vi "background4.vi"() -> ()   [LabVIEW 2014]
uses:
  cloud.ctl
  heart.ctl
  <vilib>/Utility/inputDevices.llb/keyboardAcquire.vi
  <vilib>/Utility/inputDevices.llb/closeKeyboard.vi
panel:
  out "User 1":T1
  out "User 2":T1
  out "Ring 6":T2
  out "Ring 5":T3
  out "Ring 4":T3
  out "Ring 3":T2
  out "2jump":bool=TRUE
  out "User2 name":string
  out "User1 name":string
  out "人1生命":dbl
  out "人2生命":dbl
  out "heart 6":T4
  out "heart 5":T4
  out "heart 4":T4
  out "heart 3":T4
  out "heart 2":T4
  out "heart 1":T4
  out "雲  3":T5
  out "black hole":T6
  out "雲 2":T5
  out "雲":T5
  out "1jump":bool=TRUE
  out "火右飛 2":bool=TRUE
  out "火左飛 2":bool
  out "火左飛":bool
  out "1":T7
  out "火右飛":bool=TRUE
  out "2":T8
  out "2-1":T7
  out "2-2":T8
  in  "stop jump2":bool
  in  "stop jump1":bool
  out "keys pressed":T9(array[ring])
  in  "right/left 2":bool
  in  "人2":bool
  in  "right/left":bool
  in  "人1":bool
  in  "整個遊戲中止":bool
  # "587"
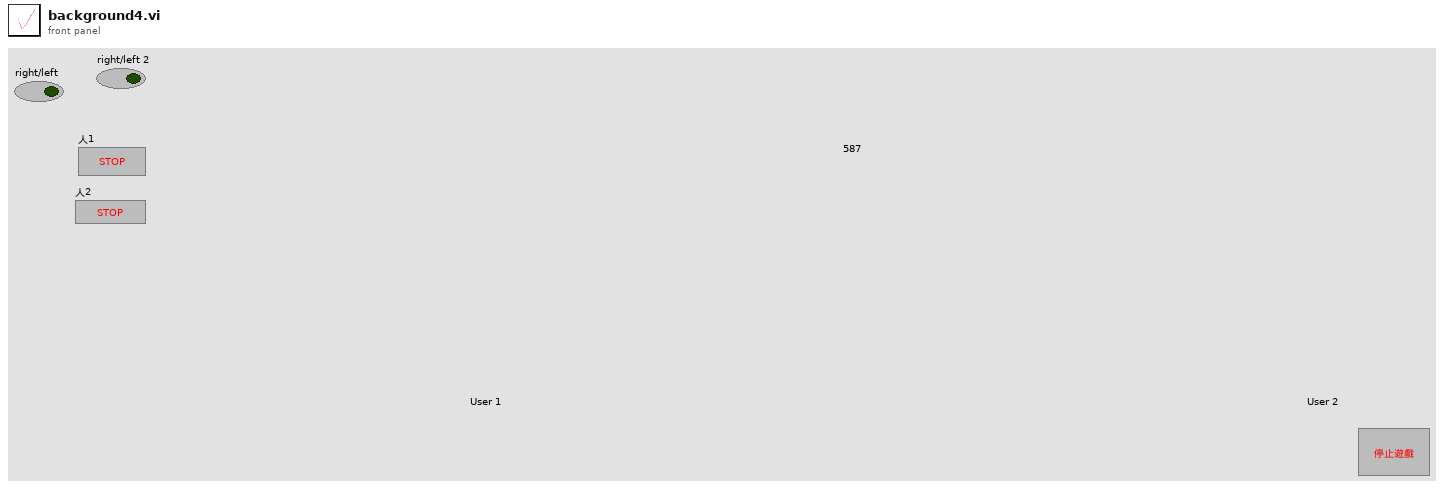
[diagram p1: front panel]
types:
  T1 = typedef "Control 3.ctl" = u16
  T2 = typedef "窄短cloud.ctl" = u16
  T3 = typedef "窄cloud.ctl" = u16
  T4 = typedef "heart.ctl" = u16
  T5 = typedef "cloud.ctl" = u16
  T6 = typedef "Control 4.ctl" = u16
  T7 = typedef "火焰.ctl" = u16
  T8 = typedef "火焰2.ctl" = u16
  T9 = enum16{"0", "1", "2", "3", "4", "5", "6", "7", "8", "9", "A", "B", "C", "D", "E", "F", "G", "H", "I", "J", "K", "L", "M", "N", "O", "P", "Q", "R", "S", "T", "U", "V", "W", "X", "Y", "Z", "F1", "F2", "F3", "F4", "F5", "F6", "F7", "F8", "F9", "F10", "F11", "F12", "F13", "F14", "F15", "ADD", "BACK", "BACKSLASH", "CAPITAL", "COMMA", "DECIMAL", "DELETE", "DIVIDE", "DOWN", "END", "EQUALS", "ESCAPE", "GRAVE (`)", "HOME", "INSERT", "LBRACKET", "LCONTROL", "LEFT", "L ALT", "LSHIFT", "LWIN", "MINUS", "MULTIPLY", "NEXT", "NUMLOCK", "NUMPAD_0", "NUMPAD_1", "NUMPAD_2", "NUMPAD_3", "NUMPAD_4", "NUMPAD_5", "NUMPAD_6", "NUMPAD_7", "NUMPAD_8", "NUMPAD_9", "PAUSE", "PERIOD", "PRIOR (PG UP)", "RBRACKET", "RCONTROL", "RETURN", "RIGHT", "R ALT", "RSHIFT", "RWIN", "SCROLL", "SEMICOLON", "SLASH", "SPACE", "SUBTRACT", "TAB", "UP", "ENTER (num pad)", "' (quote)"}[]
  T10 = enum16{"0", "1", "2", "3", "4", "5", "6", "7", "8", "9", "A", "B", "C", "D", "E", "F", "G", "H", "I", "J", "K", "L", "M", "N", "O", "P", "Q", "R", "S", "T", "U", "V", "W", "X", "Y", "Z", "F1", "F2", "F3", "F4", "F5", "F6", "F7", "F8", "F9", "F10", "F11", "F12", "F13", "F14", "F15", "ADD", "BACK", "BACKSLASH", "CAPITAL", "COMMA", "DECIMAL", "DELETE", "DIVIDE", "DOWN", "END", "EQUALS", "ESCAPE", "GRAVE (`)", "HOME", "INSERT", "LBRACKET", "LCONTROL", "LEFT", "L ALT", "LSHIFT", "LWIN", "MINUS", "MULTIPLY", "NEXT", "NUMLOCK", "NUMPAD_0", "NUMPAD_1", "NUMPAD_2", "NUMPAD_3", "NUMPAD_4", "NUMPAD_5", "NUMPAD_6", "NUMPAD_7", "NUMPAD_8", "NUMPAD_9", "PAUSE", "PERIOD", "PRIOR (PG UP)", "RBRACKET", "RCONTROL", "RETURN", "RIGHT", "R ALT", "RSHIFT", "RWIN", "SCROLL", "SEMICOLON", "SLASH", "SPACE", "SUBTRACT", "TAB", "UP", "ENTER (num pad)", "' (quote)"}
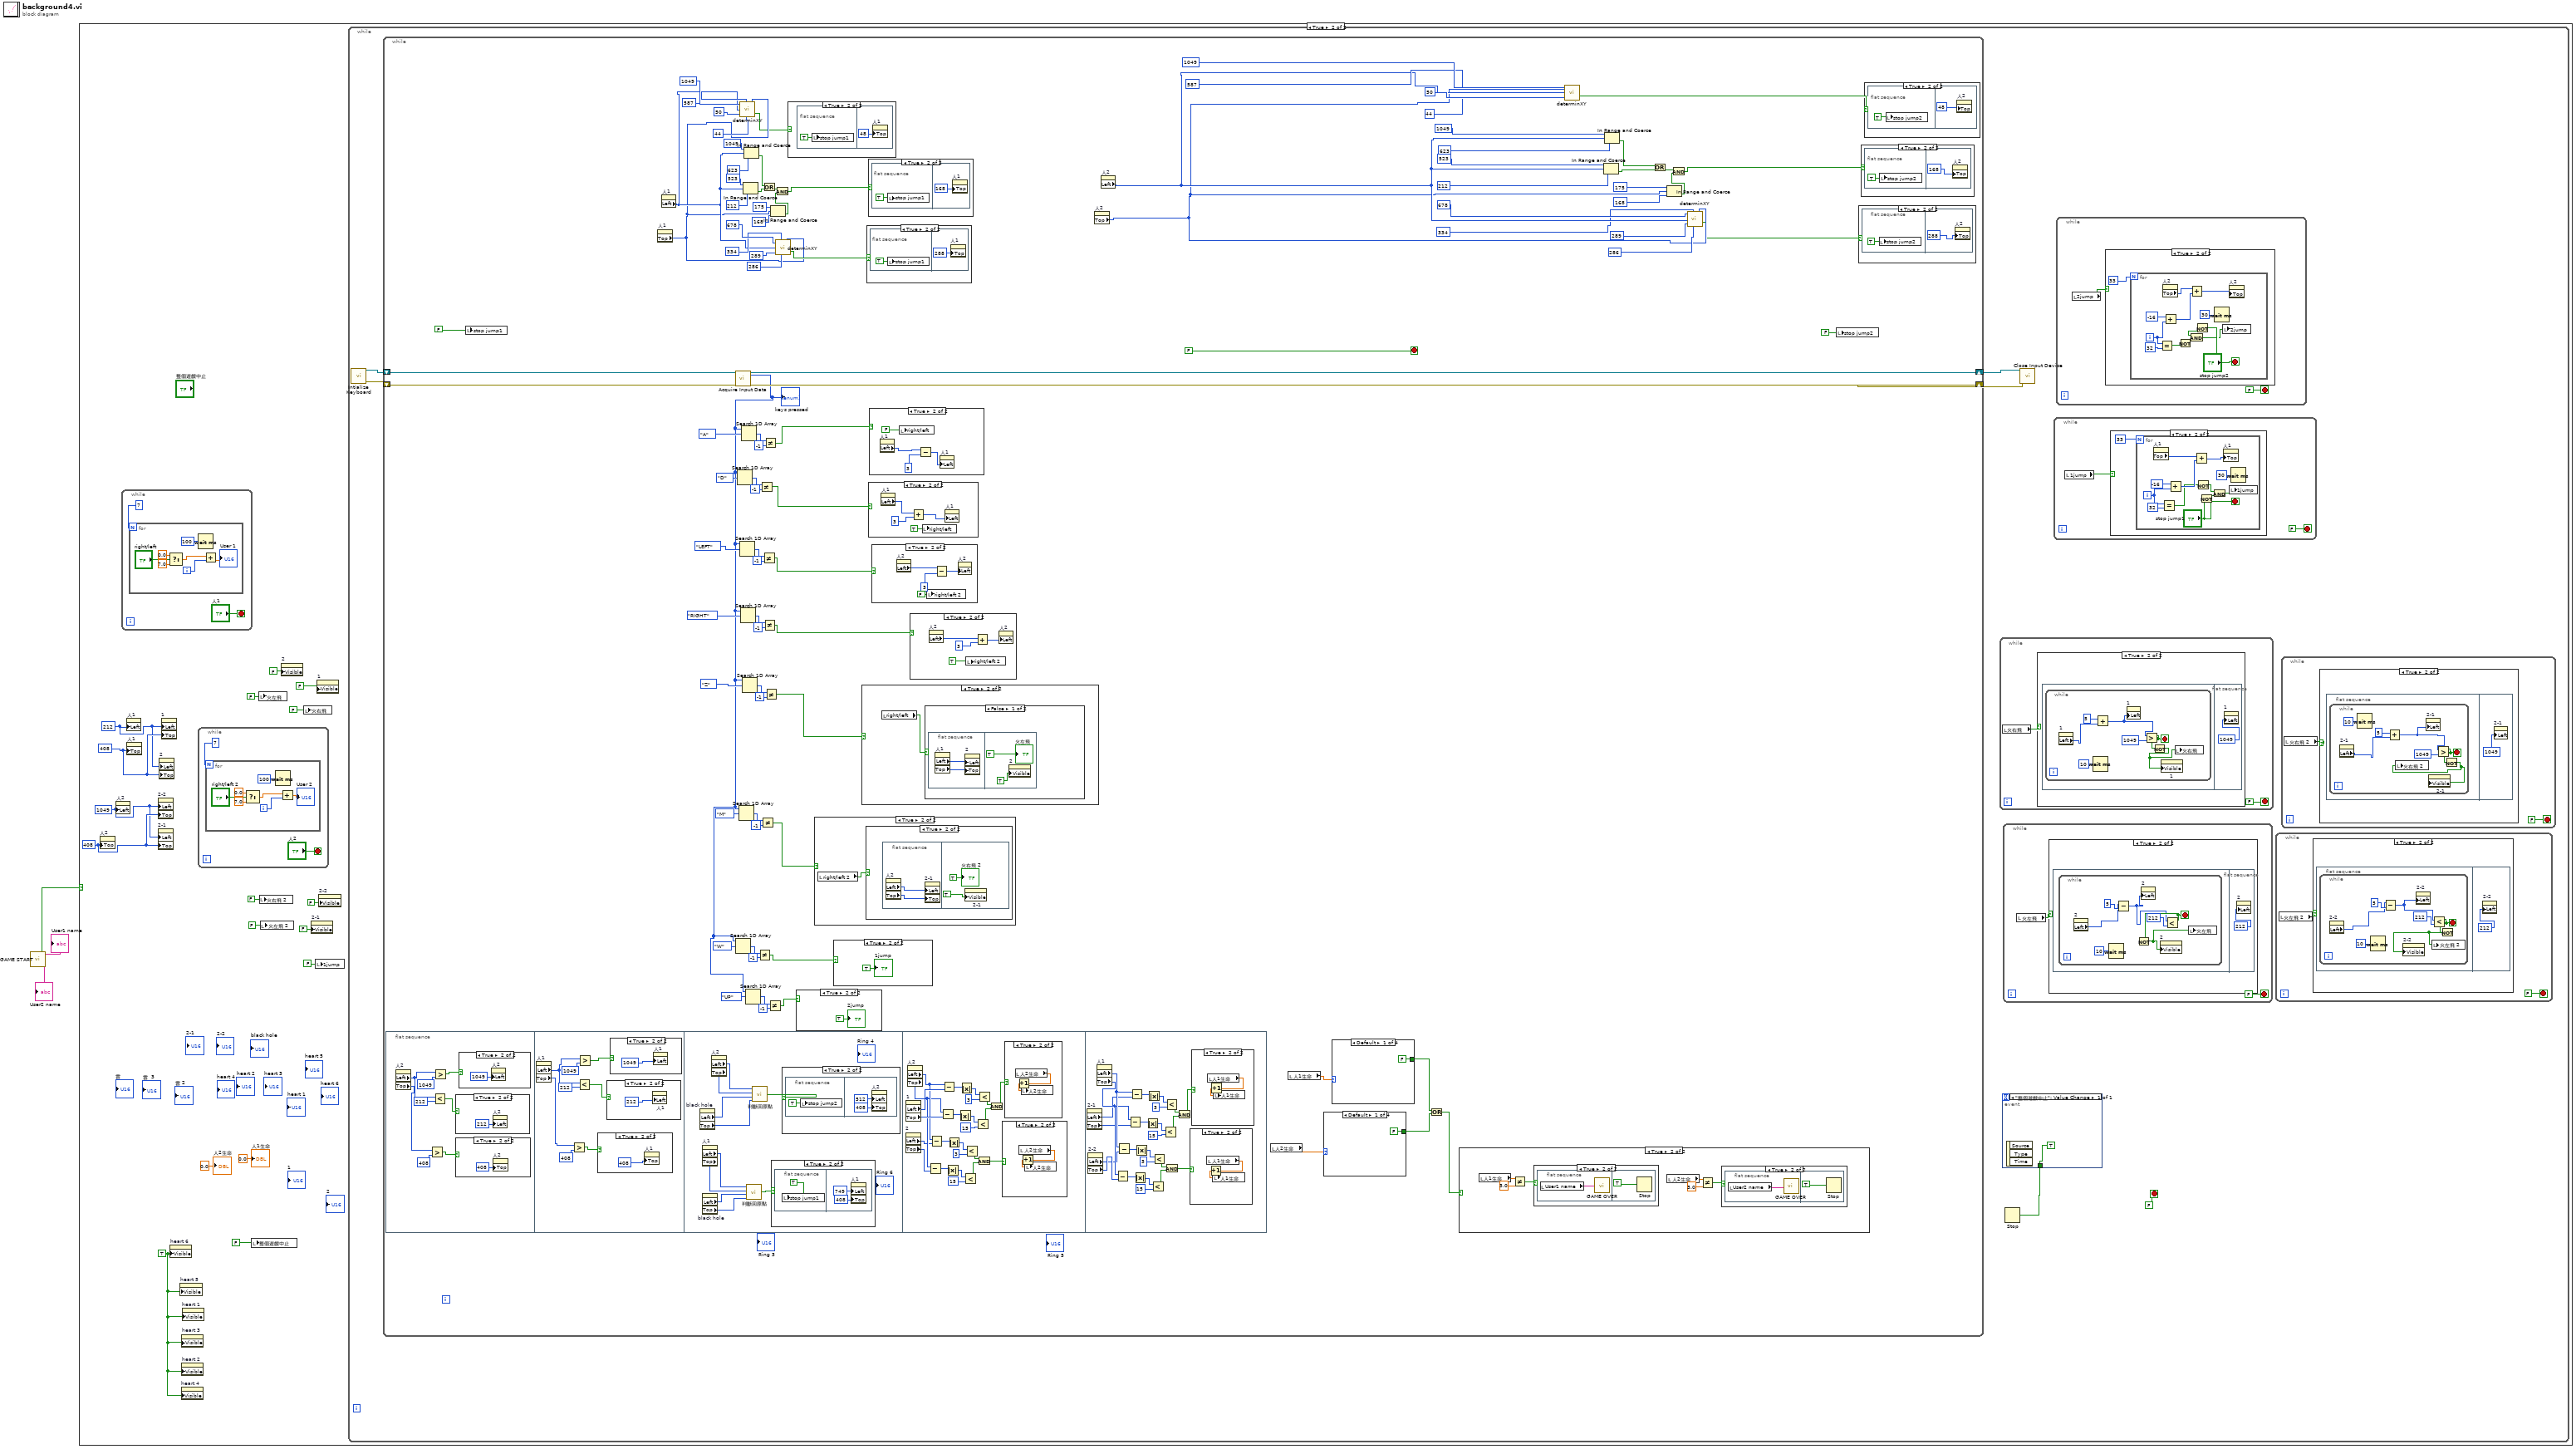
[diagram p0: block diagram]
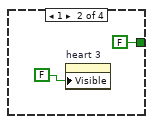
[diagram p13: hidden frame]
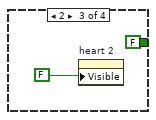
[diagram p14: hidden frame]
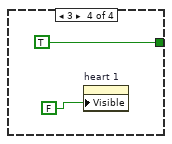
[diagram p15: hidden frame]
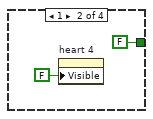
[diagram p16: hidden frame]
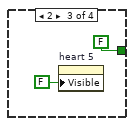
[diagram p17: hidden frame]
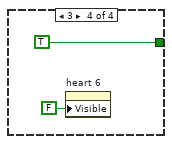
[diagram p18: hidden frame]
diagram:
  n1 = call "GAME START.vi"() -> ("stop 2"=w3:bool, "User2 name 2"=→"User2 name":string, "User1 name 2"=→"User1 name":string)  [unwired: 1 in]
  n2 = case shown="True" w3 {
    frame False {
    }
    frame True {
      w4 = TRUE ("Visible")
      w15 = 408 ("Position:Top")
      w14 = 1049 ("Position:Left")
      w13 = 408 ("Position:Top")
      w12 = 212 ("Position:Left")
      n3 = property on="人2" class="Ring (strict)"("Top"=w15) -> ()  [unwired: 2 in, 2 out]
      n4 = property on="人2" class="Ring (strict)"("Left"=w14) -> ()  [unwired: 2 in, 2 out]
      n5 = while {
        stop <- "人1" stop-if-true
        n6 = for {
          N: 7 -> [_]
          i -> [w28]
          n7 = Select(t=0.0, s="right/left", f=7.0) -> (s? t:f=w25:dbl)
          n8 = Wait (ms)(milliseconds to wait=u32 100) -> ()  [unwired: 1 out]
          n9 = Add(x=w25, y=w28) -> (x+y=→"User 1":dbl)
        }
      }
      n10 = property on="人1" class="Ring (strict)"("Left"=w12) -> ()  [unwired: 2 in, 2 out]
      n11 = property on="人1" class="Ring (strict)"("Top"=w13) -> ()  [unwired: 2 in, 2 out]
      n12 = property on="2-2" class="Ring (strict)"("Left"=w14, "Top"=w15) -> ()  [unwired: 2 in, 2 out]
      n13 = property on="2-1" class="Ring (strict)"("Left"=w14, "Top"=w15) -> ()  [unwired: 2 in, 2 out]
      n14 = property on="2" class="Ring (strict)"("Left"=w12, "Top"=w13) -> ()  [unwired: 2 in, 2 out]
      n15 = property on="1" class="Ring (strict)"("Left"=w12, "Top"=w13) -> ()  [unwired: 2 in, 2 out]
      n16 = property on="heart 6" class="Ring (strict)"("Visible"=w4) -> ()  [unwired: 2 in, 2 out]
      n17 = property on="heart 5" class="Ring (strict)"("Visible"=w4) -> ()  [unwired: 2 in, 2 out]
      n18 = property on="heart 4" class="Ring (strict)"("Visible"=w4) -> ()  [unwired: 2 in, 2 out]
      n19 = property on="heart 3" class="Ring (strict)"("Visible"=w4) -> ()  [unwired: 2 in, 2 out]
      n20 = property on="heart 2" class="Ring (strict)"("Visible"=w4) -> ()  [unwired: 2 in, 2 out]
      n21 = property on="heart 1" class="Ring (strict)"("Visible"=w4) -> ()  [unwired: 2 in, 2 out]
      n22 = while {
        stop <- "人2" stop-if-true
        n23 = for {
          N: 7 -> [_]
          i -> [w37]
          n24 = Select(t=0.0, s="right/left 2", f=7.0) -> (s? t:f=w35:dbl)
          n25 = Wait (ms)(milliseconds to wait=u32 100) -> ()  [unwired: 1 out]
          n26 = Add(x=w35, y=w37) -> (x+y=→"User 2":dbl)
        }
      }
      n27 = local write "整個遊戲中止"(FALSE ("整個遊戲中止")) -> ()
      n28 = local write "火左飛"(FALSE ("火左飛")) -> ()
      n29 = local write "火右飛 2"(FALSE ("火右飛 2")) -> ()
      n30 = local write "火左飛 2"(FALSE ("火左飛 2")) -> ()
      n31 = property on="2" class="Ring (strict)"("Visible"=FALSE) -> ()  [unwired: 2 in, 2 out]
      n32 = local write "火右飛"(FALSE ("Boolean")) -> ()
      n33 = property on="2-1" class="Ring (strict)"("Visible"=FALSE) -> ()  [unwired: 2 in, 2 out]
      n34 = local write "1jump"(FALSE ("1jump")) -> ()
      n35 = property on="1" class="Ring (strict)"("Visible"=FALSE) -> ()  [unwired: 2 in, 2 out]
      n36 = property on="2-2" class="Ring (strict)"("Visible"=FALSE) -> ()  [unwired: 2 in, 2 out]
      n37 = while {
        stop <- FALSE stop-if-true
        n38 = call <vilib>:"Intialize Keyboard.vi"() -> ("error out"=w43:errorcluster, "device ID"=w44:refnum<k1>)  [unwired: 10 in]
        n39 = while {
          shift-right: [w206] -> w41
          shift-left: w44 -> [w203]
          shift-right: [w205] -> w42
          shift-left: w43 -> [w204]
          stop <- FALSE stop-if-true
          n40 = flat-sequence {
            frame #0 {
              n41 = property on="人2" class="Ring (strict)"() -> ("Left"=w238:i32, "Top"=w233:i32)  [unwired: 2 in, 2 out]
              n42 = Greater?(x=w233, y=408) -> (0:w232:bool)
              n43 = Less?(x=w238, y=212) -> (x < y?=w235:bool)
              n44 = Greater?(x=w238, y=1049) -> (0:w236:bool)
              n45 = case shown="True" w235 {
                frame False {
                }
                frame True {
                  n46 = property on="人2" class="Ring (strict)"("Left"=212 ("Position:Left")) -> ()  [unwired: 2 in, 2 out]
                }
              }
              n47 = case shown="True" w232 {
                frame False {
                }
                frame True {
                  n48 = property on="人2" class="Ring (strict)"("Top"=408 ("Position:Left")) -> ()  [unwired: 2 in, 2 out]
                }
              }
              n49 = case shown="True" w236 {
                frame False {
                }
                frame True {
                  n50 = property on="人2" class="Ring (strict)"("Left"=1049 ("Position:Left")) -> ()  [unwired: 2 in, 2 out]
                }
              }
            }
            frame #1 {
              n51 = property on="人1" class="Ring (strict)"() -> ("Left"=w250:i32, "Top"=w243:i32)  [unwired: 2 in, 2 out]
              n52 = Greater?(x=w243, y=408) -> (0:w245:bool)
              n53 = Less?(x=w250, y=212) -> (x < y?=w249:bool)
              n54 = Greater?(x=w250, y=1049) -> (0:w248:bool)
              n55 = case shown="True" w245 {
                frame False {
                }
                frame True {
                  n56 = property on="人1" class="Ring (strict)"("Top"=408 ("Position:Left")) -> ()  [unwired: 2 in, 2 out]
                }
              }
              n57 = case shown="True" w249 {
                frame False {
                }
                frame True {
                  n58 = property on="人1" class="Ring (strict)"("Left"=212 ("Position:Left")) -> ()  [unwired: 2 in, 2 out]
                }
              }
              n59 = case shown="True" w248 {
                frame False {
                }
                frame True {
                  n60 = property on="人1" class="Ring (strict)"("Left"=1049 ("Position:Left")) -> ()  [unwired: 2 in, 2 out]
                }
              }
            }
            frame #2 {
              n61 = property on="black hole" class="Ring (strict)"() -> ("Left"=w261:i32, "Top"=w260:i32)  [unwired: 2 in, 2 out]
              n62 = property on="人1" class="Ring (strict)"() -> ("Left"=w254:i32, "Top"=w255:i32)  [unwired: 2 in, 2 out]
              n63 = property on="black hole" class="Ring (strict)"() -> ("Left"=w256:i32, "Top"=w257:i32)  [unwired: 2 in, 2 out]
              n64 = property on="人2" class="Ring (strict)"() -> ("Left"=w263:i32, "Top"=w262:i32)  [unwired: 2 in, 2 out]
              n65 = call "判斷回原點.vi"("¬}y"=w257, "¬}x"=w256, "人y"=w255, "人x"=w254) -> ("x .and. y?"=w258:bool)
              n66 = call "判斷回原點.vi"("¬}y"=w260, "¬}x"=w261, "人y"=w262, "人x"=w263) -> ("x .and. y?"=w259:bool)
              n67 = case shown="True" w258 {
                frame False {
                }
                frame True {
                  n68 = flat-sequence {
                    frame #0 {
                      n69 = local write "stop jump1"(TRUE) -> ()
                    }
                    frame #1 {
                      n70 = property on="人1" class="Ring (strict)"("Left"=749 ("Position:Left"), "Top"=408 ("Position:Top")) -> ()  [unwired: 2 in, 2 out]
                    }
                  }
                }
              }
              n71 = case shown="True" w259 {
                frame False {
                }
                frame True {
                  n72 = flat-sequence {
                    frame #0 {
                      n73 = local write "stop jump2"(TRUE ("stop jump2")) -> ()
                    }
                    frame #1 {
                      n74 = property on="人2" class="Ring (strict)"("Left"=512 ("Position:Left"), "Top"=408 ("Position:Top")) -> ()  [unwired: 2 in, 2 out]
                    }
                  }
                }
              }
            }
            frame #3 {
              n75 = property on="2" class="Ring (strict)"() -> ("Left"=w271:i32, "Top"=w270:i32)  [unwired: 2 in, 2 out]
              n76 = property on="1" class="Ring (strict)"() -> ("Left"=w293:i32, "Top"=w286:i32)  [unwired: 2 in, 2 out]
              n77 = property on="人2" class="Ring (strict)"() -> ("Left"=w273:i32, "Top"=w272:i32)  [unwired: 2 in, 2 out]
              n78 = Subtract(x=w272, y=w270) -> (x-y=w280:i32)
              n79 = Subtract(x=w273, y=w271) -> (x-y=w275:i32)
              n80 = Subtract(x=w272, y=w286) -> (x-y=w287:i32)
              n81 = Subtract(x=w273, y=w293) -> (x-y=w292:i32)
              n82 = Absolute Value(x=w280) -> (abs(x)=w279:i32)
              n83 = Absolute Value(x=w275) -> (abs(x)=w276:i32)
              n84 = Absolute Value(x=w287) -> (abs(x)=w288:i32)
              n85 = Absolute Value(x=w292) -> (abs(x)=w291:i32)
              n86 = Less?(x=w279, y=15) -> (x < y?=w282:bool)
              n87 = Less?(x=w276, y=3) -> (x < y?=w281:bool)
              n88 = Less?(x=w288, y=15) -> (x < y?=w284:bool)
              n89 = Less?(x=w291, y=3) -> (x < y?=w285:bool)
              n90 = And(x=w281, y=w282) -> (x .and. y?=w274:bool)
              n91 = And(x=w285, y=w284) -> (x .and. y?=w283:bool)
              n92 = case shown="True" w274 {
                frame False {
                }
                frame True {
                  n93 = local read "人2生命"() -> (w295:dbl)
                  n94 = Increment(x=w295) -> (x+1=w294:dbl)
                  n95 = local write "人2生命"(w294) -> ()
                }
              }
              n96 = case shown="True" w283 {
                frame False {
                }
                frame True {
                  n97 = local read "人2生命"() -> (w296:dbl)
                  n98 = Increment(x=w296) -> (x+1=w297:dbl)
                  n99 = local write "人2生命"(w297) -> ()
                }
              }
            }
            frame #4 {
              n100 = property on="2-1" class="Ring (strict)"() -> ("Left"=w300:i32, "Top"=w301:i32)  [unwired: 2 in, 2 out]
              n101 = property on="2-2" class="Ring (strict)"() -> ("Left"=w298:i32, "Top"=w299:i32)  [unwired: 2 in, 2 out]
              n102 = property on="人1" class="Ring (strict)"() -> ("Left"=w303:i32, "Top"=w302:i32)  [unwired: 2 in, 2 out]
              n103 = Subtract(x=w302, y=w299) -> (x-y=w315:i32)
              n104 = Subtract(x=w303, y=w298) -> (x-y=w320:i32)
              n105 = Subtract(x=w302, y=w301) -> (x-y=w309:i32)
              n106 = Subtract(x=w303, y=w300) -> (x-y=w304:i32)
              n107 = Absolute Value(x=w315) -> (abs(x)=w316:i32)
              n108 = Absolute Value(x=w320) -> (abs(x)=w319:i32)
              n109 = Absolute Value(x=w309) -> (abs(x)=w308:i32)
              n110 = Absolute Value(x=w304) -> (abs(x)=w305:i32)
              n111 = Less?(x=w316, y=15) -> (x < y?=w313:bool)
              n112 = Less?(x=w319, y=3) -> (x < y?=w314:bool)
              n113 = Less?(x=w308, y=15) -> (x < y?=w311:bool)
              n114 = Less?(x=w305, y=3) -> (x < y?=w310:bool)
              n115 = And(x=w314, y=w313) -> (x .and. y?=w321:bool)
              n116 = And(x=w310, y=w311) -> (x .and. y?=w312:bool)
              n117 = case shown="True" w321 {
                frame False {
                }
                frame True {
                  n118 = local read "人1生命"() -> (w323:dbl)
                  n119 = Increment(x=w323) -> (x+1=w322:dbl)
                  n120 = local write "人1生命"(w322) -> ()
                }
              }
              n121 = case shown="True" w312 {
                frame False {
                }
                frame True {
                  n122 = local read "人1生命"() -> (w324:dbl)
                  n123 = Increment(x=w324) -> (x+1=w325:dbl)
                  n124 = local write "人1生命"(w325) -> ()
                }
              }
            }
          }
          n125 = local write "stop jump1"(FALSE ("stop jump1")) -> ()
          n126 = property on="人1" class="Ring (strict)"() -> ("Top"=w139:i32)  [unwired: 2 in, 2 out]
          n127 = property on="人1" class="Ring (strict)"() -> ("Left"=w142:i32)  [unwired: 2 in, 2 out]
          n128 = call-poly <vilib>:"Acquire Input Data.vi"("device ID"=w203, "error in (no error)"=w204) -> ("device ID"=w206:refnum<k1>, "keys pressed"=w117:T9, "error out"=w205:errorcluster)  [unwired: 15 in]
          "keys pressed" <- w117
          n129 = Search 1D Array(1D array=w117, element=T10."W") -> (index of element=w152:i32)  [unwired: 1 in]
          n130 = Search 1D Array(1D array=w117, element=T10."D") -> (index of element=w197:i32)  [unwired: 1 in]
          n131 = Search 1D Array(1D array=w117, element=T10."M") -> (index of element=w159:i32)  [unwired: 1 in]
          n132 = call "determinXY.vi"("x max"=1049 ("upper limit"), "x min"=587 ("lower limit"), "x"=w142, "y max"=50 ("upper limit"), "y min"=44 ("lower limit"), "y"=w139) -> ("result"=w138:bool)
          n133 = Search 1D Array(1D array=w117, element=T10."LEFT") -> (index of element=w194:i32)  [unwired: 1 in]
          n134 = Search 1D Array(1D array=w117, element=T10."RIGHT") -> (index of element=w190:i32)  [unwired: 1 in]
          n135 = Search 1D Array(1D array=w117, element=T10."A") -> (index of element=w200:i32)  [unwired: 1 in]
          n136 = Search 1D Array(1D array=w117, element=T10."Z") -> (index of element=w162:i32)  [unwired: 1 in]
          n137 = In Range and Coerce(upper limit=523, x=w142, lower limit=212) -> (In Range?=w177:bool)  [unwired: 1 out]
          n138 = In Range and Coerce(upper limit=1049, x=w142, lower limit=623) -> (In Range?=w178:bool)  [unwired: 1 out]
          n139 = Search 1D Array(1D array=w117, element=T10."UP") -> (index of element=w119:i32)  [unwired: 1 in]
          n140 = Not Equal?(x=w152, y=-1) -> (x != y?=w150:bool)
          n141 = Not Equal?(x=w197, y=-1) -> (x != y?=w155:bool)
          n142 = Not Equal?(x=w159, y=-1) -> (x != y?=w157:bool)
          n143 = Not Equal?(x=w194, y=-1) -> (x != y?=w192:bool)
          n144 = Or(x=w178, y=w177) -> (x .or. y?=w179:bool)
          n145 = Not Equal?(x=w190, y=-1) -> (x != y?=w188:bool)
          n146 = Not Equal?(x=w200, y=-1) -> (x != y?=w156:bool)
          n147 = Not Equal?(x=w162, y=-1) -> (x != y?=w154:bool)
          n148 = Not Equal?(x=w119, y=-1) -> (x != y?=w116:bool)
          n149 = In Range and Coerce(upper limit=175, x=w139, lower limit=168 ("y")) -> (In Range?=w183:bool)  [unwired: 1 out]
          n150 = And(x=w179, y=w183) -> (x .and. y?=w176:bool)
          n151 = call "determinXY.vi"("x max"=678 ("upper limit"), "x min"=334 ("lower limit"), "x"=w142, "y max"=289 ("upper limit"), "y min"=286 ("y"), "y"=w139) -> ("result"=w145:bool)
          n152 = case shown="True" w138 {
            frame False {
            }
            frame True {
              n153 = flat-sequence {
                frame #0 {
                  n154 = local write "stop jump1"(TRUE ("stop jump1")) -> ()
                }
                frame #1 {
                  n155 = property on="人1" class="Ring (strict)"("Top"=48 ("Position:Top")) -> ()  [unwired: 2 in, 2 out]
                }
              }
            }
          }
          n156 = case shown="True" w116 {
            frame False {
            }
            frame True {
              "2jump" <- TRUE ("2jump")
            }
          }
          n157 = case shown="True" w157 {
            frame False {
            }
            frame True {
              n158 = local read "right/left 2"() -> (w327:bool)
              n159 = case shown="True" w327 {
                frame False {
                  n160 = flat-sequence {
                    frame #0 {
                      n161 = property on="人2" class="Ring (strict)"() -> ("Left"=w329:i32, "Top"=w328:i32)  [unwired: 2 in, 2 out]
                      n162 = property on="2-2" class="Ring (strict)"("Left"=w329, "Top"=w328) -> ()  [unwired: 2 in, 2 out]
                    }
                    frame #1 {
                      n163 = property on="2-2" class="Ring (strict)"("Visible"=TRUE) -> ()  [unwired: 2 in, 2 out]
                      "火左飛 2" <- TRUE
                    }
                  }
                }
                frame True {
                  n164 = flat-sequence {
                    frame #0 {
                      n165 = property on="人2" class="Ring (strict)"() -> ("Left"=w333:i32, "Top"=w332:i32)  [unwired: 2 in, 2 out]
                      n166 = property on="2-1" class="Ring (strict)"("Left"=w333, "Top"=w332) -> ()  [unwired: 2 in, 2 out]
                    }
                    frame #1 {
                      n167 = property on="2-1" class="Ring (strict)"("Visible"=TRUE) -> ()  [unwired: 2 in, 2 out]
                      "火右飛 2" <- TRUE
                    }
                  }
                }
              }
            }
          }
          n168 = case shown="True" w150 {
            frame False {
            }
            frame True {
              "1jump" <- TRUE
            }
          }
          n169 = case shown="True" w154 {
            frame False {
            }
            frame True {
              n170 = local read "right/left"() -> (w336:bool)
              n171 = case shown="False" w336 {
                frame False {
                  n172 = flat-sequence {
                    frame #0 {
                      n173 = property on="人1" class="Ring (strict)"() -> ("Left"=w338:i32, "Top"=w337:i32)  [unwired: 2 in, 2 out]
                      n174 = property on="2" class="Ring (strict)"("Left"=w338, "Top"=w337) -> ()  [unwired: 2 in, 2 out]
                    }
                    frame #1 {
                      n175 = property on="2" class="Ring (strict)"("Visible"=TRUE) -> ()  [unwired: 2 in, 2 out]
                      "火左飛" <- TRUE
                    }
                  }
                }
                frame True {
                  n176 = flat-sequence {
                    frame #0 {
                      n177 = property on="人1" class="Ring (strict)"() -> ("Left"=w342:i32, "Top"=w341:i32)  [unwired: 2 in, 2 out]
                      n178 = property on="1" class="Ring (strict)"("Left"=w342, "Top"=w341) -> ()  [unwired: 2 in, 2 out]
                    }
                    frame #1 {
                      n179 = property on="1" class="Ring (strict)"("Visible"=TRUE) -> ()  [unwired: 2 in, 2 out]
                      "火右飛" <- TRUE
                    }
                  }
                }
              }
            }
          }
          n180 = case shown="True" w145 {
            frame False {
            }
            frame True {
              n181 = flat-sequence {
                frame #0 {
                  n182 = local write "stop jump1"(TRUE ("stop jump1")) -> ()
                }
                frame #1 {
                  n183 = property on="人1" class="Ring (strict)"("Top"=288 ("Position:Top")) -> ()  [unwired: 2 in, 2 out]
                }
              }
            }
          }
          n184 = case shown="True" w176 {
            frame False {
            }
            frame True {
              n185 = flat-sequence {
                frame #0 {
                  n186 = local write "stop jump1"(TRUE ("stop jump1")) -> ()
                }
                frame #1 {
                  n187 = property on="人1" class="Ring (strict)"("Top"=168 ("Position:Top")) -> ()  [unwired: 2 in, 2 out]
                }
              }
            }
          }
          n188 = case shown="True" w155 {
            frame False {
            }
            frame True {
              n189 = property on="人1" class="Ring (strict)"() -> ("Left"=w367:i32)  [unwired: 2 in, 2 out]
              n190 = Add(x=w367, y=3) -> (x+y=w366:i32)
              n191 = local write "right/left"(TRUE ("right/left")) -> ()
              n192 = property on="人1" class="Ring (strict)"("Left"=w366) -> ()  [unwired: 2 in, 2 out]
            }
          }
          n193 = case shown="True" w156 {
            frame False {
            }
            frame True {
              n194 = property on="人1" class="Ring (strict)"() -> ("Left"=w370:i32)  [unwired: 2 in, 2 out]
              n195 = local write "right/left"(FALSE ("人1 right 2")) -> ()
              n196 = Subtract(x=w370, y=3) -> (x-y=w369:i32)
              n197 = property on="人1" class="Ring (strict)"("Left"=w369) -> ()  [unwired: 2 in, 2 out]
            }
          }
          n198 = case shown="True" w192 {
            frame False {
            }
            frame True {
              n199 = property on="人2" class="Ring (strict)"() -> ("Left"=w363:i32)  [unwired: 2 in, 2 out]
              n200 = local write "right/left 2"(FALSE ("right/left")) -> ()
              n201 = Subtract(x=w363, y=3) -> (x-y=w362:i32)
              n202 = property on="人2" class="Ring (strict)"("Left"=w362) -> ()  [unwired: 2 in, 2 out]
            }
          }
          n203 = case shown="True" w188 {
            frame False {
            }
            frame True {
              n204 = property on="人2" class="Ring (strict)"() -> ("Left"=w359:i32)  [unwired: 2 in, 2 out]
              n205 = local write "right/left 2"(TRUE ("人1 right 2")) -> ()
              n206 = Add(x=w359, y=3) -> (x+y=w358:i32)
              n207 = property on="人2" class="Ring (strict)"("Left"=w358) -> ()  [unwired: 2 in, 2 out]
            }
          }
          n208 = property on="人2" class="Ring (strict)"() -> ("Top"=w127:i32)  [unwired: 2 in, 2 out]
          n209 = property on="人2" class="Ring (strict)"() -> ("Left"=w131:i32)  [unwired: 2 in, 2 out]
          n210 = local read "人2生命"() -> (w125:dbl)
          n211 = local read "人1生命"() -> (w124:dbl)
          n212 = case shown="Default" w125 {
            tunnel: [FALSE ("整個遊戲中止") FALSE ("整個遊戲中止") FALSE ("整個遊戲中止") TRUE ("整個遊戲中止")] -> w122
            frame Default {
            }
            frame 1 {
              n213 = property on="heart 4" class="Ring (strict)"("Visible"=FALSE) -> ()  [unwired: 2 in, 2 out]
            }
            frame 2 {
              n214 = property on="heart 5" class="Ring (strict)"("Visible"=FALSE) -> ()  [unwired: 2 in, 2 out]
            }
            frame 3 {
              n215 = property on="heart 6" class="Ring (strict)"("Visible"=FALSE) -> ()  [unwired: 2 in, 2 out]
            }
          }
          n216 = case shown="Default" w124 {
            tunnel: [FALSE ("整個遊戲中止") FALSE ("整個遊戲中止") FALSE ("整個遊戲中止") TRUE ("整個遊戲中止")] -> w123
            frame Default {
            }
            frame 1 {
              n217 = property on="heart 3" class="Ring (strict)"("Visible"=FALSE) -> ()  [unwired: 2 in, 2 out]
            }
            frame 2 {
              n218 = property on="heart 2" class="Ring (strict)"("Visible"=FALSE) -> ()  [unwired: 2 in, 2 out]
            }
            frame 3 {
              n219 = property on="heart 1" class="Ring (strict)"("Visible"=FALSE) -> ()  [unwired: 2 in, 2 out]
            }
          }
          n220 = Or(x=w123, y=w122) -> (x .or. y?=w121:bool)
          n221 = case shown="True" w121 {
            frame False {
            }
            frame True {
              n222 = local read "人1生命"() -> (w213:dbl)
              n223 = Not Equal?(x=w213, y=3.0) -> (x != y?=w211:bool)
              n224 = case shown="True" w211 {
                frame False {
                }
                frame True {
                  n225 = flat-sequence {
                    frame #0 {
                      n226 = local read "User1 name"() -> (w216:string)
                      n227 = call "GAME OVER.vi"("name"=w216) -> ()  [unwired: 1 in]
                    }
                    frame #1 {
                      n228 = Stop(stop? (T)=TRUE) -> ()
                    }
                  }
                }
              }
              n229 = local read "人2生命"() -> (w208:dbl)
              n230 = Not Equal?(x=w208, y=3.0) -> (x != y?=w210:bool)
              n231 = case shown="True" w210 {
                frame False {
                }
                frame True {
                  n232 = flat-sequence {
                    frame #0 {
                      n233 = local read "User2 name"() -> (w214:string)
                      n234 = call "GAME OVER.vi"("name"=w214) -> ()  [unwired: 1 in]
                    }
                    frame #1 {
                      n235 = Stop(stop? (T)=TRUE) -> ()
                    }
                  }
                }
              }
            }
          }
          n236 = call "determinXY.vi"("x max"=1049 ("upper limit"), "x min"=587 ("lower limit"), "x"=w131, "y max"=50 ("upper limit"), "y min"=44 ("lower limit"), "y"=w127) -> ("result"=w133:bool)
          n237 = In Range and Coerce(upper limit=523, x=w131, lower limit=212) -> (In Range?=w166:bool)  [unwired: 1 out]
          n238 = In Range and Coerce(upper limit=1049, x=w131, lower limit=623) -> (In Range?=w167:bool)  [unwired: 1 out]
          n239 = Or(x=w167, y=w166) -> (x .or. y?=w168:bool)
          n240 = In Range and Coerce(upper limit=175, x=w127, lower limit=168 ("y")) -> (In Range?=w171:bool)  [unwired: 1 out]
          n241 = And(x=w168, y=w171) -> (x .and. y?=w165:bool)
          n242 = call "determinXY.vi"("x max"=678 ("upper limit"), "x min"=334 ("lower limit"), "x"=w131, "y max"=289 ("upper limit"), "y min"=286 ("y"), "y"=w127) -> ("result"=w126:bool)
          n243 = local write "stop jump2"(FALSE ("stop jump1 2")) -> ()
          n244 = case shown="True" w126 {
            frame False {
            }
            frame True {
              n245 = flat-sequence {
                frame #0 {
                  n246 = local write "stop jump2"(TRUE ("stop jump1")) -> ()
                }
                frame #1 {
                  n247 = property on="人2" class="Ring (strict)"("Top"=288 ("Position:Top")) -> ()  [unwired: 2 in, 2 out]
                }
              }
            }
          }
          n248 = case shown="True" w165 {
            frame False {
            }
            frame True {
              n249 = flat-sequence {
                frame #0 {
                  n250 = local write "stop jump2"(TRUE ("stop jump1")) -> ()
                }
                frame #1 {
                  n251 = property on="人2" class="Ring (strict)"("Top"=168 ("Position:Top")) -> ()  [unwired: 2 in, 2 out]
                }
              }
            }
          }
          n252 = case shown="True" w133 {
            frame False {
            }
            frame True {
              n253 = flat-sequence {
                frame #0 {
                  n254 = local write "stop jump2"(TRUE ("stop jump1")) -> ()
                }
                frame #1 {
                  n255 = property on="人2" class="Ring (strict)"("Top"=48 ("Position:Top")) -> ()  [unwired: 2 in, 2 out]
                }
              }
            }
          }
        }
        n256 = while {
          stop <- FALSE stop-if-true
          n257 = local read "火右飛"() -> (w82:bool)
          n258 = case shown="True" w82 {
            frame False {
            }
            frame True {
              n259 = flat-sequence {
                frame #0 {
                  n260 = while {
                    stop <- w87 stop-if-true
                    n261 = property on="1" class="Ring (strict)"() -> ("Left"=w86:i32)  [unwired: 2 in, 2 out]
                    n262 = Wait (ms)(milliseconds to wait=u32 10) -> ()  [unwired: 1 out]
                    n263 = Add(x=5, y=w86) -> (x+y=w85:i32)
                    n264 = property on="1" class="Ring (strict)"("Left"=w85) -> ()  [unwired: 2 in, 2 out]
                    n265 = Greater?(x=w85, y=1049) -> (0:w87:bool)
                    n266 = Not(x=w87) -> (.not. x?=w83:bool)
                    n267 = property on="1" class="Ring (strict)"("Visible"=w83) -> ()  [unwired: 2 in, 2 out]
                    n268 = local write "火右飛"(w83) -> ()
                  }
                }
                frame #1 {
                  n269 = property on="1" class="Ring (strict)"("Left"=1049 ("y")) -> ()  [unwired: 2 in, 2 out]
                }
              }
            }
          }
        }
        n270 = event shown="[0] \"整個遊戲中止\": Value Change" {
          selector: _ -> [_]
          dyn-events: _ -> [_]
          timeout: _ -> [_]
          tunnel: [TRUE] -> w40
          event "整個遊戲中止": Value Change {
            n271 = event-data() -> ()  [unwired: 1 in, 3 out]
          }
        }
        n272 = while {
          stop <- FALSE stop-if-true
          n273 = local read "火左飛"() -> (w92:bool)
          n274 = case shown="True" w92 {
            frame False {
            }
            frame True {
              n275 = flat-sequence {
                frame #0 {
                  n276 = while {
                    stop <- w99 stop-if-true
                    n277 = property on="2" class="Ring (strict)"() -> ("Left"=w97:i32)  [unwired: 2 in, 2 out]
                    n278 = Wait (ms)(milliseconds to wait=u32 10) -> ()  [unwired: 1 out]
                    n279 = Subtract(x=w97, y=5 ("x")) -> (x-y=w94:i32)
                    n280 = property on="2" class="Ring (strict)"("Left"=w94) -> ()  [unwired: 2 in, 2 out]
                    n281 = Less?(x=w94, y=212) -> (x < y?=w99:bool)
                    n282 = Not(x=w99) -> (.not. x?=w93:bool)
                    n283 = property on="2" class="Ring (strict)"("Visible"=w93) -> ()  [unwired: 2 in, 2 out]
                    n284 = local write "火左飛"(w93) -> ()
                  }
                }
                frame #1 {
                  n285 = property on="2" class="Ring (strict)"("Left"=212 ("y")) -> ()  [unwired: 2 in, 2 out]
                }
              }
            }
          }
        }
        n286 = Stop(stop? (T)=w40) -> ()
        n287 = call-poly <vilib>:"Close Input Device.vi"("error in (no error)"=w42, "device ID"=w41) -> ()  [unwired: 8 in, 1 out]
        n288 = while {
          stop <- FALSE stop-if-true
          n289 = local read "1jump"() -> (w46:bool)
          n290 = case shown="True" w46 {
            frame False {
            }
            frame True {
              n291 = for {
                N: 33 -> [_]
                i -> [w54]
                stop <- "stop jump1" stop-if-true
                n292 = property on="人1" class="Ring (strict)"() -> ("Top"=w57:i32)  [unwired: 2 in, 2 out]
                n293 = Equal?(x=w54, y=32) -> (x = y?=w52:bool)
                n294 = Add(x=-16, y=w54) -> (x+y=w59:i32)
                n295 = Add(x=w57, y=w59) -> (x+y=w56:i32)
                n296 = Not(x=w52) -> (.not. x?=w51:bool)
                n297 = Not(x="stop jump1") -> (.not. x?=w50:bool)
                n298 = And(x=w51, y=w50) -> (x .and. y?=w49:bool)
                n299 = property on="人1" class="Ring (strict)"("Top"=w56) -> ()  [unwired: 2 in, 2 out]
                n300 = local write "1jump"(w49) -> ()
                n301 = Wait (ms)(milliseconds to wait=u32 30) -> ()  [unwired: 1 out]
              }
            }
          }
        }
        n302 = while {
          stop <- FALSE stop-if-true
          n303 = local read "2jump"() -> (w101:bool)
          n304 = case shown="True" w101 {
            frame False {
            }
            frame True {
              n305 = for {
                N: 33 -> [_]
                i -> [w109]
                stop <- "stop jump2" stop-if-true
                n306 = Equal?(x=w109, y=32) -> (x = y?=w108:bool)
                n307 = property on="人2" class="Ring (strict)"() -> ("Top"=w112:i32)  [unwired: 2 in, 2 out]
                n308 = Add(x=-16, y=w109) -> (x+y=w114:i32)
                n309 = Not(x=w108) -> (.not. x?=w107:bool)
                n310 = Add(x=w112, y=w114) -> (x+y=w111:i32)
                n311 = Not(x="stop jump2") -> (.not. x?=w106:bool)
                n312 = And(x=w106, y=w107) -> (x .and. y?=w104:bool)
                n313 = Wait (ms)(milliseconds to wait=u32 30) -> ()  [unwired: 1 out]
                n314 = local write "2jump"(w104) -> ()
                n315 = property on="人2" class="Ring (strict)"("Top"=w111) -> ()  [unwired: 2 in, 2 out]
              }
            }
          }
        }
        n316 = while {
          stop <- FALSE stop-if-true
          n317 = local read "火左飛 2"() -> (w62:bool)
          n318 = case shown="True" w62 {
            frame False {
            }
            frame True {
              n319 = flat-sequence {
                frame #0 {
                  n320 = while {
                    stop <- w69 stop-if-true
                    n321 = property on="2-2" class="Ring (strict)"() -> ("Left"=w67:i32)  [unwired: 2 in, 2 out]
                    n322 = Wait (ms)(milliseconds to wait=u32 10) -> ()  [unwired: 1 out]
                    n323 = Subtract(x=w67, y=5 ("x")) -> (x-y=w64:i32)
                    n324 = property on="2-2" class="Ring (strict)"("Left"=w64) -> ()  [unwired: 2 in, 2 out]
                    n325 = Less?(x=w64, y=212) -> (x < y?=w69:bool)
                    n326 = Not(x=w69) -> (.not. x?=w63:bool)
                    n327 = property on="2-2" class="Ring (strict)"("Visible"=w63) -> ()  [unwired: 2 in, 2 out]
                    n328 = local write "火左飛 2"(w63) -> ()
                  }
                }
                frame #1 {
                  n329 = property on="2-2" class="Ring (strict)"("Left"=212 ("y")) -> ()  [unwired: 2 in, 2 out]
                }
              }
            }
          }
        }
        n330 = while {
          stop <- FALSE stop-if-true
          n331 = local read "火右飛 2"() -> (w72:bool)
          n332 = case shown="True" w72 {
            frame False {
            }
            frame True {
              n333 = flat-sequence {
                frame #0 {
                  n334 = while {
                    stop <- w77 stop-if-true
                    n335 = property on="2-1" class="Ring (strict)"() -> ("Left"=w76:i32)  [unwired: 2 in, 2 out]
                    n336 = Wait (ms)(milliseconds to wait=u32 10) -> ()  [unwired: 1 out]
                    n337 = Add(x=5, y=w76) -> (x+y=w75:i32)
                    n338 = property on="2-1" class="Ring (strict)"("Left"=w75) -> ()  [unwired: 2 in, 2 out]
                    n339 = Greater?(x=w75, y=1049) -> (0:w77:bool)
                    n340 = Not(x=w77) -> (.not. x?=w73:bool)
                    n341 = local write "火右飛 2"(w73) -> ()
                    n342 = property on="2-1" class="Ring (strict)"("Visible"=w73) -> ()  [unwired: 2 in, 2 out]
                  }
                }
                frame #1 {
                  n343 = property on="2-1" class="Ring (strict)"("Left"=1049 ("y")) -> ()  [unwired: 2 in, 2 out]
                }
              }
            }
          }
        }
      }
      "人2生命" <- 0.0 ("人1生命")
      "人1生命" <- 0.0 ("人2生命")
    }
  }
